vi "CallOpenCVLib.vi"(8 "error in (no error)":errorcluster, 9 "Eyes Cascade Path":path, 10 "Face Cascade Path":path, 11 "Image Src":T2) -> (0 "error out":errorcluster, 1 "Eyes":T1[](array[typedef]) {"Rotation" format="%.2f"; "Left" scale=0.0..1024.0; "Right" scale=0.0..1024.0}, 2 "Faces":T1[](array[typedef]) {"Rotation" format="%.2f"; "Left" scale=0.0..1024.0; "Right" scale=0.0..1024.0}, 3 "Image Dst Out":T2)   [LabVIEW 2019]
doc: "<b> NIVisOpenCV FaceDetection</b> is a sample VI to use OpenCV Face Detection algorithm"
uses:
  <vilib>/vision/Image Controls.llb/IMAQ Image.ctl
  nivisocvsamples.dll
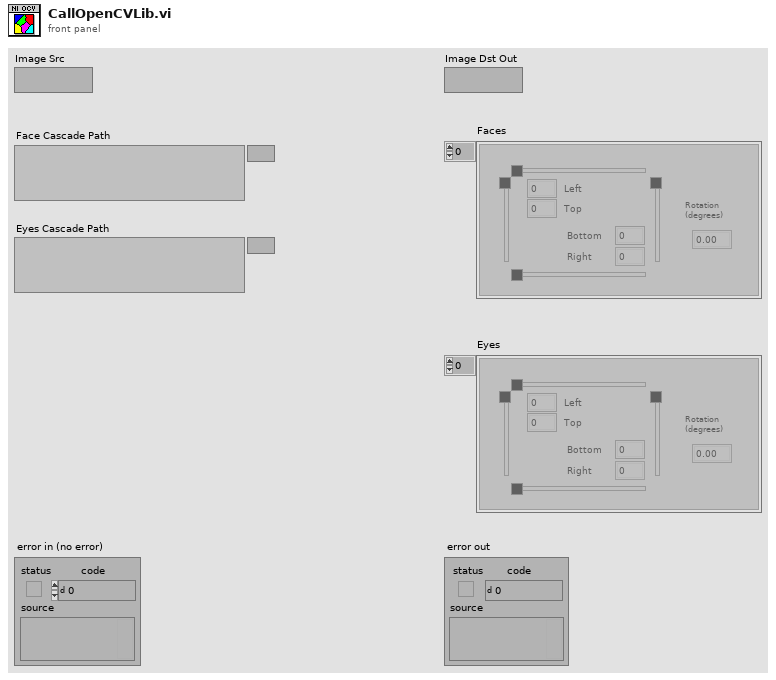
[diagram p1: front panel]
types:
  T1 = typedef "IMAQ Rectangle" = cluster{"Left":i32, "Top":i32, "Right":i32, "Bottom":i32, "Rotation":dbl}
  T2 = typedef "IMAQ Image.ctl" = refnum<image>
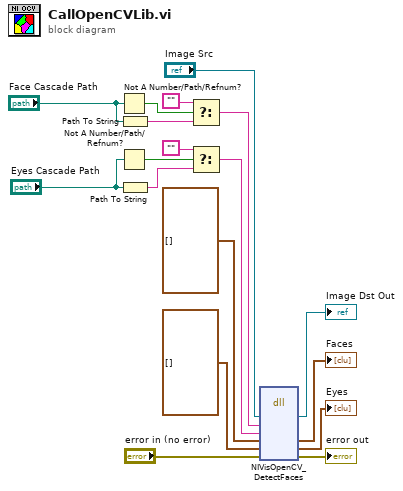
[diagram p0: block diagram]
diagram:
  n1 = Not A Number/Path/Refnum?(number/path/refnum="Face Cascade Path") -> (NaN/Path/Refnum?=w6:bool)
  n2 = Not A Number/Path/Refnum?(number/path/refnum="Eyes Cascade Path") -> (NaN/Path/Refnum?=w13:bool)
  n3 = Path To String(path="Face Cascade Path") -> (string=w8:string)
  n4 = Path To String(path="Eyes Cascade Path") -> (string=w10:string)
  n5 = Select(t="", s=w6, f=w8) -> (s? t:f=w5:string)
  n6 = Select(t="", s=w13, f=w10) -> (s? t:f=w9:string)
  n7 = dll-call lib="nivisocvsamples.dll" fn="NIVisOpenCV_DetectFaces"("Image Src"="Image Src", "facesCascadePath"=w5, "eyesCascadePath"=w9, "faces"=T1[] [] ("Faces"), "eyes"=T1[] [] ("Eyes"), "error"="error in (no error)") -> ("Image Src"=→"Image Dst Out":T2, "faces"=→"Faces":T1[], "eyes"=→"Eyes":T1[], "error"=→"error out":errorcluster)  [unwired: 6 in, 2 out]
